vi "SubVI_ALD-Process_V16.vi"(0 "error in (no error)":errorcluster, 1 "Precursors List (Strings)":string[](array[string]), 2 "Digital Output Assignments":T7, 5 "output cluster":T3, 7 "output cluster 4":T2, 9 "Graph Ref Cluster":T4, 12 "Exec Array":dbl[][](array[numeric])) -> (4 "error out":errorcluster)   [LabVIEW 2026]
uses:
  <vilib>/Utility/miscctls.llb/LVRowAndColumnTypeDef.ctl
  <vilib>/Analysis/NI_AALBase.lvlib
  <vilib>/Analysis/baseanly.llb/Mean (DBL).vi
  CTRL_DO Boolean Array Cluster_V16.ctl
  CTRL_DO Arrays Precursor Process_V16.ctl
  CTRL_Digital-Out-Assignments_V16.ctl
panel:
  out "Total Steps":i32
  out "Summary File Refnum":refnum<file>
  in  "ProcessStep Input Cluster":T1
  out "DeltaM-i":dbl
  out "FinalMass-i":dbl
  out "InitialMass-i":dbl
  out "Dose File Refnum":refnum<file>
  out "Precursor-i name":string
  out "PrecursorValveArrays-i":T5
  out "ProcessType-i":i32
  out "PurgeTime-i":dbl
  out "DoseTime-i":dbl
  out "FillPressure-i":dbl
  out "Precursor-i":i32
  out "Delay Start Time (sec)":dbl
  out "ALD Running?":bool
  # "This VI receives the execution array and the reference cluster from the main VI to execute the ALD process. The VI first initilizes the valves to OFF, wait for the initial delay, then the VI processes the Execution Array line  by line and color each line as it is being processed. For each line of the Execution array, the VI calls the  ALDPulsePurge.vi if the Fill pressure is -1. Otherwise the ALD FHP.vi is called. There are 2 Pulse Purge processes. The Full Flow Pulse Purge process is used when the Pulse Purge Type control from the main VI is false, which indicates the Full Flow state. The Diversion Pulse Purge process is used when the Pulse Purge Type control is true. Finally, the VI returns the controls from the main VI to its original states."
  # "Module 7 Connections\nDigital Output (6V-30V)\n\n0:  Hold/Divert N2\n1:  Hold/Divert Manifold A\n2:  Hold/Divert Manifold B\n3:  Hold/Divert Manifold C\n4:  Hold/Divert Manifold D\n5:  Unused\n6:  Unused\n7:  Unused\n8:   V+ from 24V Power Supply\n9:   V- from 24V Power Supply"
  # "Module 8 Connections\nDigital Output (6V-30V)\n\n0:   Hold Chamber\n1:   Pulse A1\n2:   Pulse B1\n3:   Pulse C2\n4:   Pulse D2\n5:   Unused\n6:   Unused\n7:   Unused\n8:   V+ from 24V Power Supply\n9:   V- from 24V Power Supply"
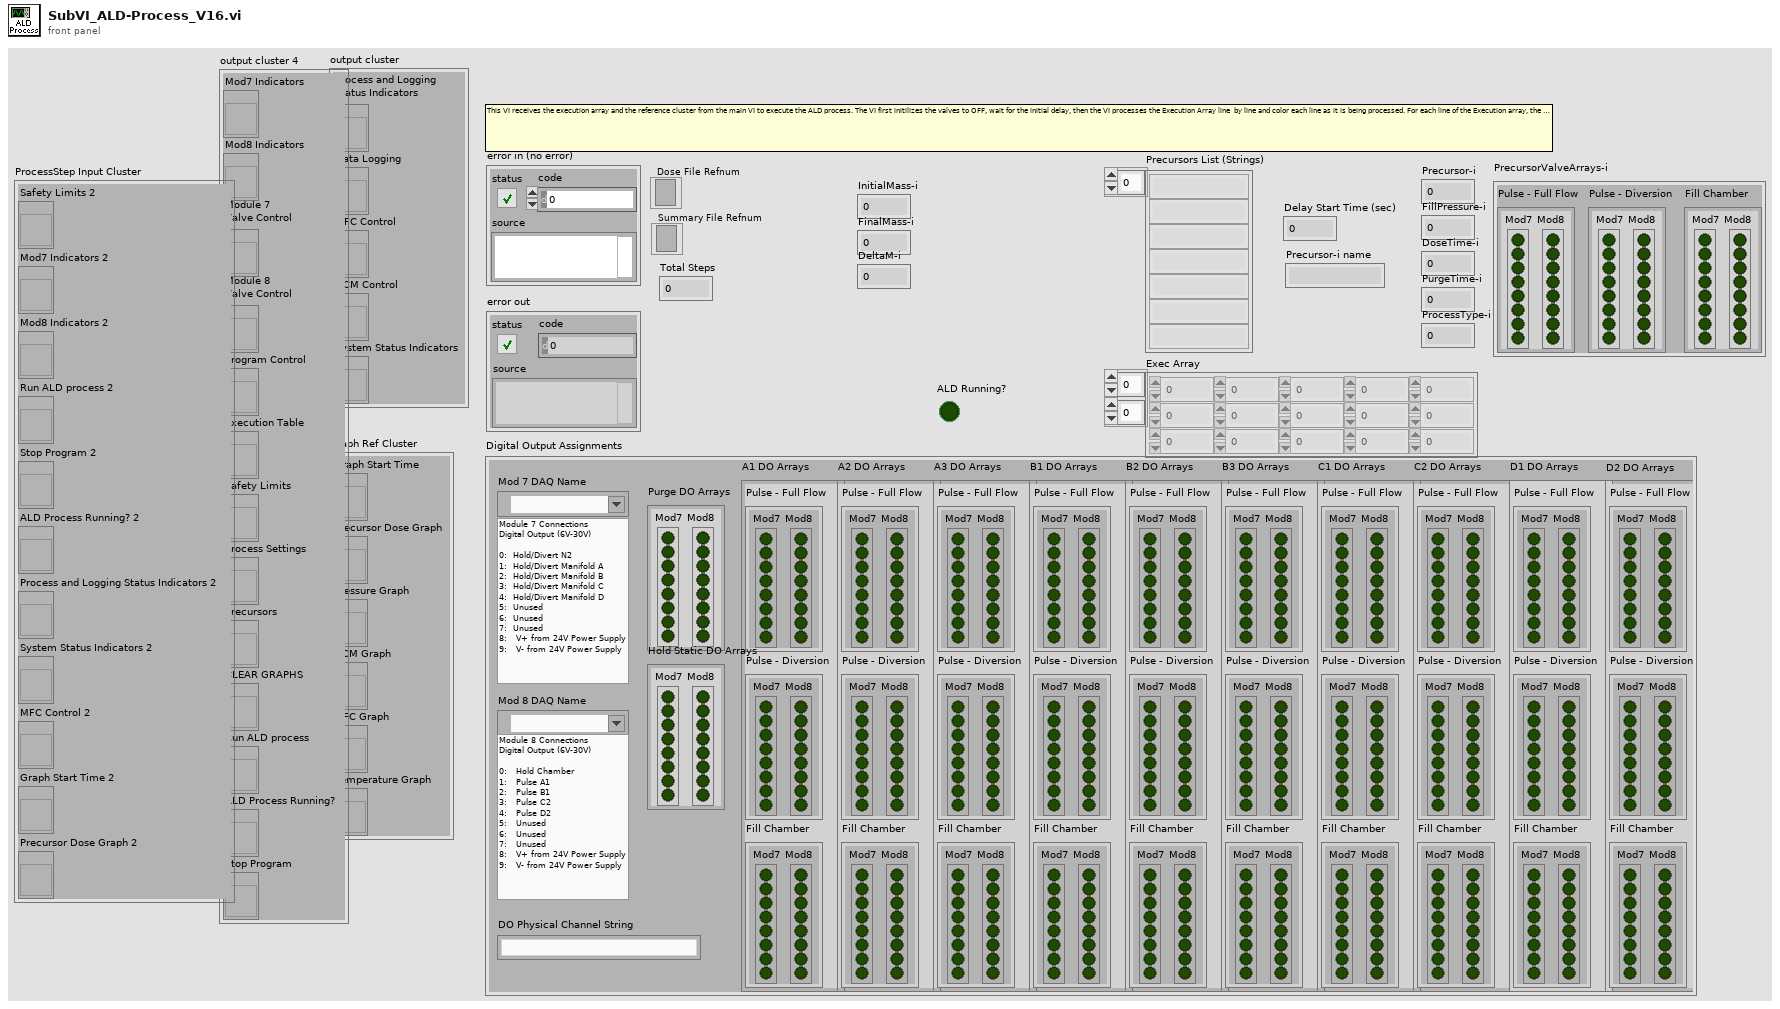
[diagram p1: front panel]
types:
  T1 = cluster{"Safety Limits 2":refnum<vi>, "Mod7 Indicators 2":refnum<vi>, "Mod8 Indicators 2":refnum<vi>, "Run ALD process 2":refnum<vi>, "Stop Program 2":refnum<vi>, "ALD Process Running? 2":refnum<vi>, "Process and Logging Status Indicators 2":refnum<vi>, "System Status Indicators 2":refnum<vi>, "MFC Control 2":refnum<vi>, "Graph Start Time 2":refnum<vi>, "Precursor Dose Graph 2":refnum<vi>}
  T2 = cluster{"Mod7 Indicators ":refnum<vi>, "Mod8 Indicators":refnum<vi>, "Module 7 \nValve Control":refnum<vi>, "Module 8 \nValve Control":refnum<vi>, "Program Control":refnum<vi>, "Execution Table":refnum<vi>, "Safety Limits":refnum<vi>, "Process Settings":refnum<vi>, "Precursors":refnum<vi>, "CLEAR GRAPHS":refnum<vi>, "Run ALD process":refnum<vi>, "ALD Process Running?":refnum<vi>, "Stop Program":refnum<vi>}
  T3 = cluster{"Process and Logging \nStatus Indicators":refnum<vi>, "Data Logging":refnum<vi>, "MFC Control":refnum<vi>, "QCM Control":refnum<vi>, "System Status Indicators":refnum<vi>}
  T4 = cluster{"Graph Start Time":refnum<vi>, "Precursor Dose Graph":refnum<vi>, "Pressure Graph":refnum<vi>, "QCM Graph":refnum<vi>, "MFC Graph":refnum<vi>, "Temperature Graph":refnum<vi>}
  T5 = typedef "CTRL_DO Arrays Precursor Process_V16.ctl" = cluster{"Pulse - Full Flow":T6, "Pulse - Diversion":T6, "Fill Chamber":T6}
  T6 = typedef "CTRL_DO Boolean Array Cluster_V16.ctl" = cluster{"Mod7":bool[], "Mod8":bool[]}
  T7 = typedef "CTRL_Digital-Out-Assignments_V16.ctl" = cluster{"Mod 7 DAQ Name":tag, "Mod 8 DAQ Name":tag, "DO Physical Channel String":string, "Purge DO Arrays":T6, "Hold Static DO Arrays":T6, "A1 DO Arrays":T5, "A2 DO Arrays":T5, "A3 DO Arrays":T5, "B1 DO Arrays":T5, "B2 DO Arrays":T5, "B3 DO Arrays":T5, "C1 DO Arrays":T5, "C2 DO Arrays":T5, "D1 DO Arrays":T5, "D2 DO Arrays":T5}
  T8 = typedef "LVRowAndColumnTypeDef.ctl" = cluster{"Row":i32, "Column":i32}
  T9 = enum16{"open", "replace", "create", "open or create", "replace or create", "replace or create with confirmation"}
  T10 = cluster{"Line 1":bool, "Line 2":bool, "Line 3":bool, "Line 4":bool, "Line 0":bool}
  T11 = cluster{"Data Log On?":bool, "User:":string, "Furnace Temp [ºC]":dbl, "Parent Directory:":path, "File Name Format:":string, "Notes:":string}
  T12 = typedef "System Status Indicators.ctl" = cluster{"System Status:":string, "Thermocouple 1":dbl, "Thermocouple 2":dbl, "Thermocouple 3":dbl, "Thermocouple 4":dbl, "Chamber Pressure (Torr)":dbl, "Pump Pressure (Torr)":dbl}
  T13 = cluster{"ALD Process Status:":string, "Logging Data to:":path, "Process Start Time:":string, "Process End Time:":string, "Steps Completed:":string}
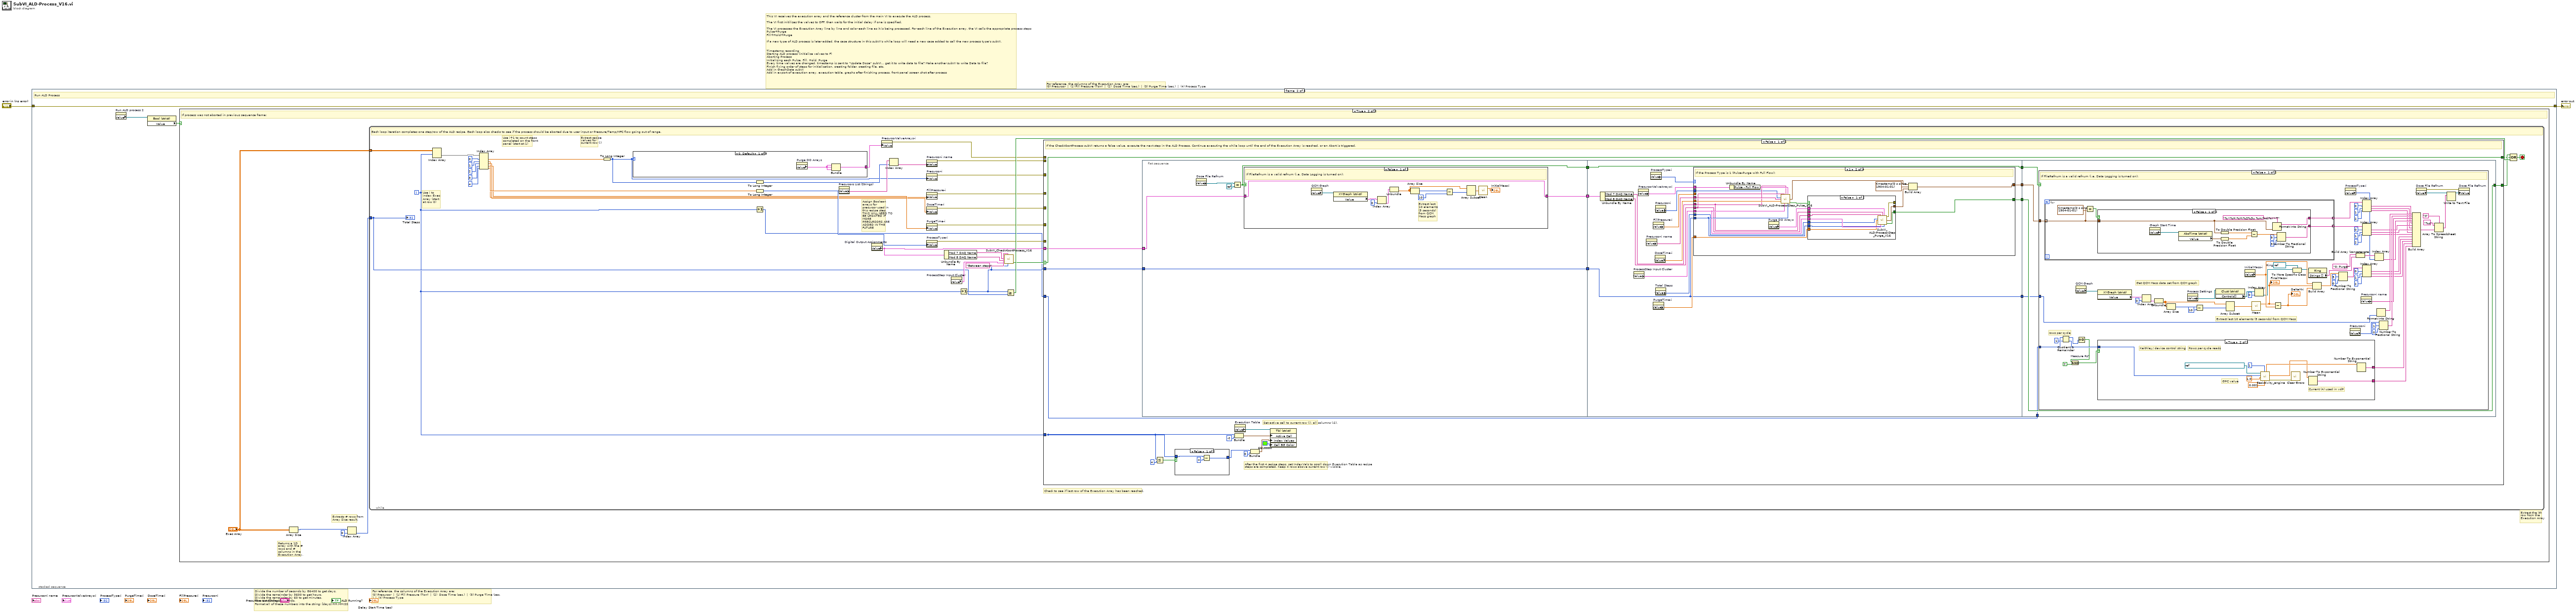
[diagram p0: block diagram]
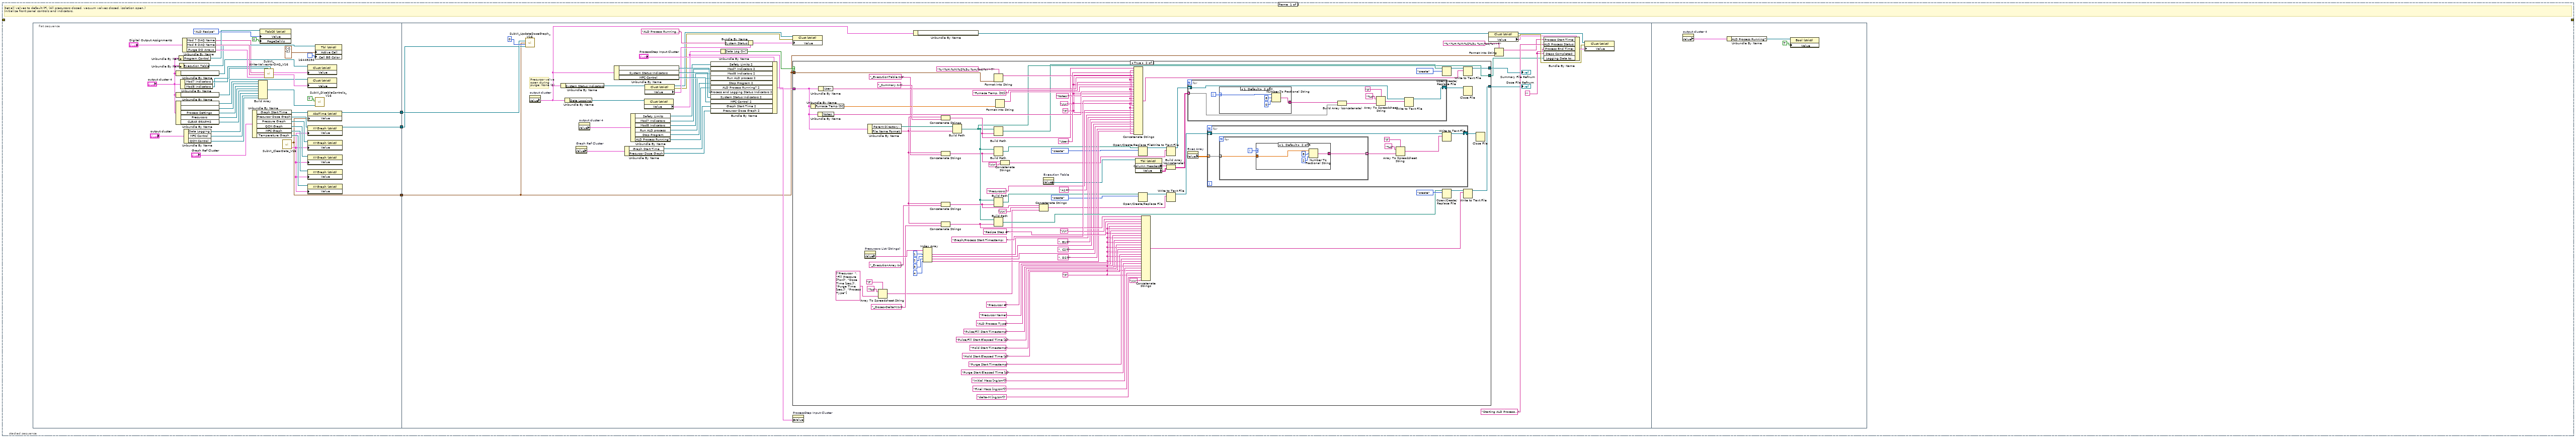
[diagram p2: hidden frame]
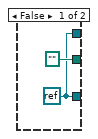
[diagram p3: hidden frame]
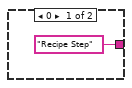
[diagram p4: hidden frame]
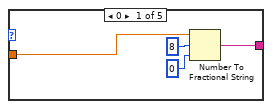
[diagram p5: hidden frame]
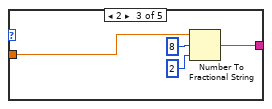
[diagram p6: hidden frame]
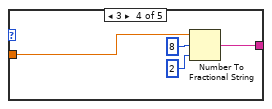
[diagram p7: hidden frame]
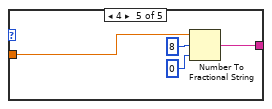
[diagram p8: hidden frame]
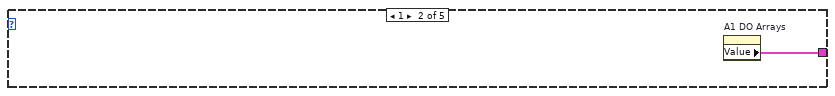
[diagram p10: hidden frame]
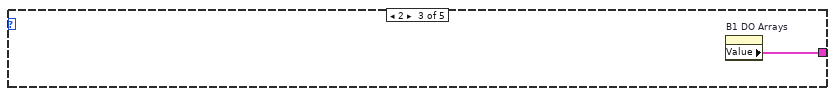
[diagram p11: hidden frame]
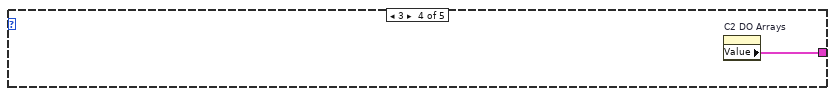
[diagram p12: hidden frame]
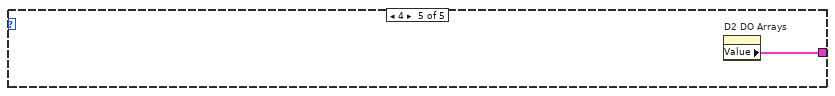
[diagram p13: hidden frame]
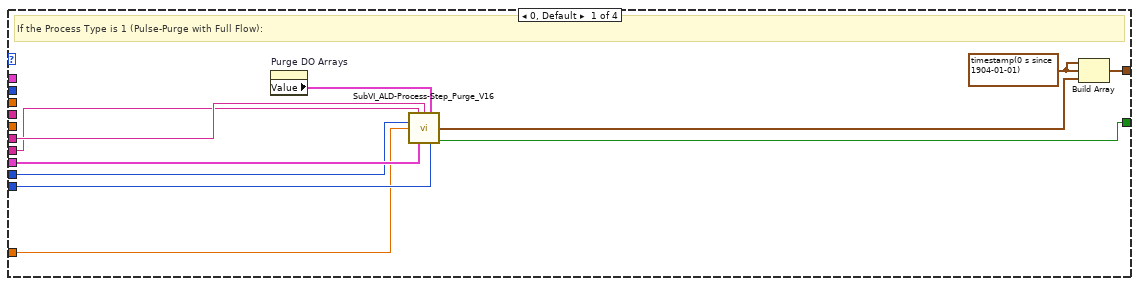
[diagram p15: hidden frame]
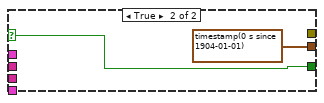
[diagram p16: hidden frame]
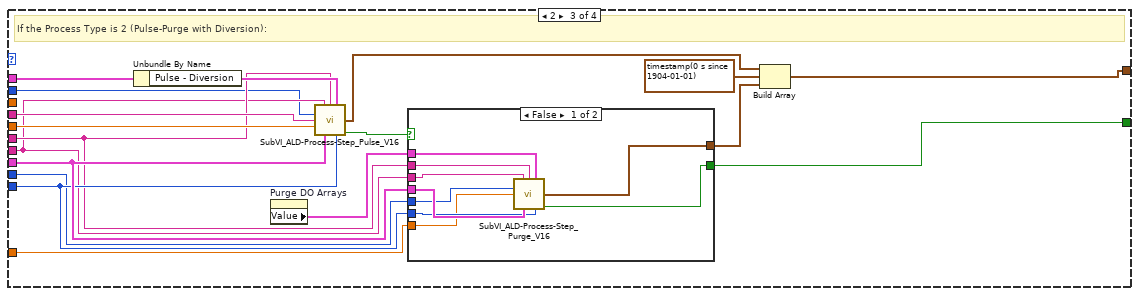
[diagram p17: hidden frame]
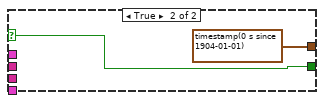
[diagram p18: hidden frame]
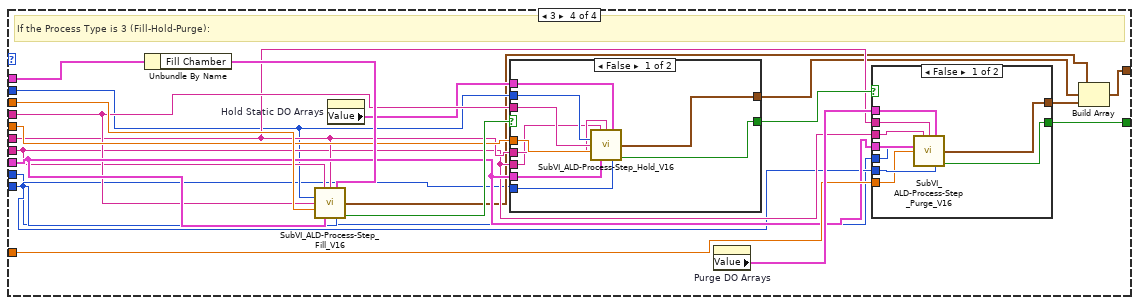
[diagram p19: hidden frame]
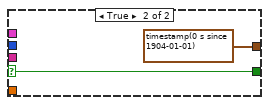
[diagram p20: hidden frame]
diagram:
  # "For reference, the columns of the Execution Array are:\n(0) Precursor  |  (1) Fill Pressure (Torr)  |  (2)  Dose Time (sec.)  |  (3) Purge Time (sec.)  |  (4) Process Type"
  # "For reference, the columns of the Execution Array are:\n(0) Precursor  |  (1) Fill Pressure (Torr)  |  (2)  Dose Time (sec.)  |  (3) Purge Time (sec.)  |  (4) Process Type"
  # "Divide the number of seconds by 86400 to get days.\nDivide the remainder by 3600 to get hours.\nDivide the remainder by 60 to get minutes.\nThe remainder is seconds.\nFormat all of these numbers into the string: [days] HH:MM:SS"
  # "This VI receives the execution array and the reference cluster from the main VI to execute the ALD process.\n\nThe VI first initilizes the valves to OFF, then waits for the initial delay if one is specified.\n\nThe VI processes the Execution Array line by line and color each line as it is being processed. For each line of the Execution array, the VI calls the appropriate process steps\nPulse+Purge\nFill+Hold+Purge\n\nIf a new type of ALD process is later added, the case structure in this subVI's while loop will need a new case added to call the new process type's subVI.\n\n\nTimestamp recording\nStarting ALD process (initialize valves to F)\nAborting Process\nInitializing each Pulse, Fill, Hold, Purge\nEvery time valves are changed, timestamp is sent to \"Update Dose\" subVI… get it to write data to file? Make another subVI to write Data to file?\nFinish fixing order of steps for initialization, creating folder, creating file, etc.\nAdd in GraphData subVI\nAdd in export of execution array, execution table, graphs after finishing process, front panel screen shot after process"
  n1 = stacked-sequence {
    tunnel: "error in (no error)" -> [_ w223 _]
    tunnel: [_ w223 _] -> w1
    frame #0 {
      # "Set all valves to default (F). (All precursors closed, vacuum valves closed, isolation open.)\nInitialize front panel controls and indicators."
      n2 = flat-sequence {
        tunnel: [w10] -> w5
        tunnel: [w9] -> w4
        tunnel: [w7] -> w3
        tunnel: w5 -> [w51]
        tunnel: w4 -> [w50]
        tunnel: w3 -> [w45]
        frame #0 {
          n3 = Unbundle By Name("output cluster 4") -> ("Module 7 \nValve Control"=w14:refnum<vi>)
          n4 = Unbundle By Name("output cluster 4") -> ("Module 8 \nValve Control"=w13:refnum<vi>)
          n5 = Unbundle By Name("output cluster 4") -> ("Module 7 \nValve Control"=w26:refnum<vi>, "Module 8 \nValve Control"=w25:refnum<vi>, "Process Settings"=w24:refnum<vi>, "Precursors"=w23:refnum<vi>, "CLEAR GRAPHS"=w22:refnum<vi>)
          n6 = Unbundle By Name("output cluster 4") -> ("Program Control"=w15:refnum<vi>)
          n7 = Unbundle By Name("output cluster 4") -> ("Execution Table"=w12:refnum<vi>)
          n8 = Unbundle By Name("output cluster 4") -> ("Mod7 Indicators"=w36:refnum<vi>, "Mod8 Indicators"=w35:refnum<vi>)
          n9 = Unbundle By Name("Digital Output Assignments") -> ("Mod 7 DAQ Name"=w6:tag, "Mod 8 DAQ Name"=w39:tag, "Purge DO Arrays"=w40:T6)
          n10 = Unbundle By Name("output cluster") -> ("Data Logging"=w21:refnum<vi>, "MFC Control"=w20:refnum<vi>, "QCM Control"=w19:refnum<vi>)
          n11 = Unbundle By Name("Graph Ref Cluster") -> ("Graph Start Time"=w34:refnum<vi>, "Precursor Dose Graph"=w33:refnum<vi>, "Pressure Graph"=w32:refnum<vi>, "QCM Graph"=w31:refnum<vi>, "MFC Graph"=w30:refnum<vi>, "Temperature Graph"=w29:refnum<vi>)
          n12 = Build Array(w26, w25, w24, w23, w22, w21, w20, w19) -> (w27:refnum<vi>[])
          n13 = property on="Property Node" class="TabCtl (strict)"(reference=w15, "Value"=enum32{"Initialization", "ALD Recipe"}."ALD Recipe", "PageSelVis"=TRUE ("Page Selector Visible")) -> ()  [unwired: 1 in, 2 out]
          n14 = call "SubVI_Write-Valves-to-DAQ_V16.vi"("Mod7 Indicators Ref"=w36, "Mod8 Indicators Ref"=w35, "DO Boolean Array Cluster"=w40, "Mod8 Port Name"=w39, "Mod7 Port Name"=w6) -> ("Mod8 Buttons"=w16:T10, "Mod7 Buttons"=w17:T10)  [unwired: 3 in, 2 out]
          n15 = call "SubVI_ClearData_V16.vi"() -> ("Time Stamp"=w7:timestamp, "Empty Graph Data"=w8:cluster{dbl[], dbl[]}[])  [unwired: 11 in, 3 out]
          n16 = property class="Clust (strict)"(reference=w14, "Value"=w17) -> ()  [unwired: 1 in, 2 out]
          n17 = property class="Clust (strict)"(reference=w13, "Value"=w16) -> ()  [unwired: 1 in, 2 out]
          n18 = property class="XYGraph (strict)"(reference=w33, "Value"=w8) -> (reference out=w9:refnum<vi>)  [unwired: 1 in, 1 out]
          n19 = property class="XYGraph (strict)"(reference=w32, "Value"=w8) -> ()  [unwired: 1 in, 2 out]
          n20 = property class="XYGraph (strict)"(reference=w31, "Value"=w8) -> ()  [unwired: 1 in, 2 out]
          n21 = property class="XYGraph (strict)"(reference=w30, "Value"=w8) -> ()  [unwired: 1 in, 2 out]
          n22 = property class="XYGraph (strict)"(reference=w29, "Value"=w8) -> ()  [unwired: 1 in, 2 out]
          n23 = property class="AbsTime (strict)"(reference=w34, "Value"=w7) -> (reference out=w10:refnum<vi>)  [unwired: 1 in, 1 out]
          n24 = property on="Property Node" class="Tbl (strict)"(reference=w12, "Active Cell"=T8 {"Row"=-2, "Column"=-2} ("Active Cell:Active Cell"), "Cell BG Color"=u32 16448250) -> ()  [unwired: 1 in, 2 out]
          n25 = call "SubVI_DisableControls_V16.vi"("appended array"=w27, "Disabled?"=TRUE) -> ()  [unwired: 9 in, 1 out]
        }
        frame #1 {
          w57 = ""
          # "Precursor valve open during purge: None (0)"
          n26 = call "SubVI_UpdateDoseGraph_V16.vi"("Graph Start Time"=w51, "New Timestamp"=w45, "Precursor Valve Open"=0 ("Precursor"), "Precursor Dose Graph"=w50) -> ()  [unwired: 11 in, 1 out]
          n27 = property on="output cluster" class="Clust (strict)"() -> ("Value"=w85:T3)  [unwired: 2 in, 2 out]
          n28 = Unbundle By Name(w85) -> ("System Status Indicators"=w55:refnum<vi>)
          n29 = Unbundle By Name(w85) -> ("Data Logging"=w68:refnum<vi>)
          n30 = property on="Graph Ref Cluster" class="Clust (strict)"() -> ("Value"=w76:T4)  [unwired: 2 in, 2 out]
          n31 = property on="output cluster 4" class="Clust (strict)"() -> ("Value"=w72:T2)  [unwired: 2 in, 2 out]
          n32 = Unbundle By Name(w85) -> ("Process and Logging \nStatus Indicators"=w80:refnum<vi>, "System Status Indicators"=w81:refnum<vi>, "MFC Control"=w82:refnum<vi>)
          n33 = Unbundle By Name(w76) -> ("Graph Start Time"=w83:refnum<vi>, "Precursor Dose Graph"=w84:refnum<vi>)
          n34 = Unbundle By Name(w72) -> ("Safety Limits"=w73:refnum<vi>, "Mod7 Indicators"=w74:refnum<vi>, "Mod8 Indicators"=w75:refnum<vi>, "Run ALD process"=w77:refnum<vi>, "Stop Program"=w78:refnum<vi>, "ALD Process Running?"=w79:refnum<vi>)
          n35 = property class="Clust (strict)"(reference=w68) -> ("Value"=w69:T11)  [unwired: 1 in, 2 out]
          n36 = property class="Clust (strict)"(reference=w55) -> (reference out=w65:refnum<vi>, error out=w64:errorcluster, "Value"=w67:T12)  [unwired: 1 in]
          n37 = Bundle By Name(cluster="ProcessStep Input Cluster", "Safety Limits 2"=w73, "Mod7 Indicators 2"=w74, "Mod8 Indicators 2"=w75, "Run ALD process 2"=w77, "Stop Program 2"=w78, "ALD Process Running? 2"=w79, "Process and Logging Status Indicators 2"=w80, "System Status Indicators 2"=w81, "MFC Control 2"=w82, "Graph Start Time 2"=w83, "Precursor Dose Graph 2"=w84) -> (w71:T1)
          n38 = Unbundle By Name(w69) -> ("Data Log On?"=w52:bool)
          n39 = Bundle By Name(cluster=w67, "System Status:"="ALD Process Running...") -> (w63:T12)
          n40 = property class="Clust (strict)"(reference=w65, error in=w64, "Value"=w63) -> ()  [unwired: 2 out]
          n41 = case shown="True" w52 {
            tunnel: [w86 w160] -> w53
            tunnel: w69 -> [_ w161]
            tunnel: w45 -> [_ w156]
            tunnel: [path "" w99] -> w48
            tunnel: [w86 w123] -> w49
            frame False {
              w86 = refnum<k0> refnum
            }
            frame True {
              w118 = "\t"
              w133 = "\t"
              w124 = "\r\n"
              n42 = Unbundle By Name(w161) -> ("Furnace Temp [ºC]"=w166:dbl)
              n43 = Unbundle By Name(w161) -> ("Notes:"=w165:string)
              n44 = Unbundle By Name(w161) -> ("User:"=w170:string)
              n45 = property on="Precursors List (Strings)" class="Arr (strict)"() -> ("Value"=w154:string[])  [unwired: 2 in, 2 out]
              n46 = Unbundle By Name(w161) -> ("Parent Directory:"=w155:path, "File Name Format:"=w98:string)
              n47 = Array To Spreadsheet String(delimiter (Tab)="\t", array=string[] ["Precursor  ", "Fill Pressure [Torr]", "Dose Time [sec.]", "Purge Time [sec.]", "Process Type"], 3:"%s" ("format string")) -> (spreadsheet string=w104:string)
              n48 = Index Array(array=w154, index #1=1 ("index"), index #2=2 ("index"), index #3=3 ("index"), index #4=4 ("index")) -> (element #1=w131:string, element #2=w129:string, element #3=w127:string, element #4=w126:string)
              n49 = Concatenate Strings(w98, "_Summary.txt" ("string")) -> (w119:string)
              n50 = Concatenate Strings(w98, "_ExecutionTable.txt" ("string")) -> (w90:string)
              n51 = Concatenate Strings(w98, "_ExecutionArray.txt" ("string")) -> (w109:string)
              n52 = Concatenate Strings(w98, "_Doses-DeltaM.txt" ("string")) -> (w136:string)
              n53 = Build Path(base path=w155, name or relative path=w98) -> (appended path=w99:path)
              n54 = Format Into String(format string="%<%H:%M:%S%3u %m/%d/%Y>T", w156) -> (resulting string=w163:string)  [unwired: 2 in, 1 out]
              n55 = Build Path(base path=w99, name or relative path=w119) -> (appended path=w139:path)
              n56 = Build Path(base path=w99, name or relative path=w90) -> (appended path=w100:path)
              n57 = Build Path(base path=w99, name or relative path=w109) -> (appended path=w115:path)
              n58 = Build Path(base path=w99, name or relative path=w136) -> (appended path=w162:path)
              n59 = Format Into String(w166) -> (resulting string=w168:string)  [unwired: 3 in, 1 out]
              n60 = Concatenate Strings(w90, "\r\n") -> (w88:string)
              n61 = Concatenate Strings(w109, "\r\n", w104) -> (w107:string)
              n62 = property on="Execution Table" class="LVObjRef (strict)"() -> ("Value"=w102:refnum<vi>)  [unwired: 2 in, 2 out]
              n63 = Concatenate Strings(w119, w124, "User:", w133, w170, w124, "Furnace Temp. [ºC]:", w133, w168, w124, "Notes:", w133, w165, w124, "Graph/Process Start Timestamp:   ", w133, w163, w124, "Precursors:", w133, "A1=", w131, ", B1=", w129, ", C2=", w127, ", D2=", w126, w124) -> (w121:string)
              n64 = property class="Tbl (strict)"(reference=w102) -> ("Column Headers[]"=w93:string[], "Value"=w92:string[][])  [unwired: 1 in, 2 out]
              n65 = Open/Create/Replace File(file path (use dialog)=w100, operation (0:open)=T9."create") -> (refnum out=w101:refnum<file>)  [unwired: 4 in, 2 out]
              n66 = Open/Create/Replace File(file path (use dialog)=w115, operation (0:open)=T9."create") -> (refnum out=w111:refnum<file>)  [unwired: 4 in, 2 out]
              n67 = Concatenate Strings(w136, "\r\n", "Recipe Step #", w118, "Precursor #", w118, "Precursor Name", w118, "ALD Process Type", w118, "Pulse/Fill Start Timestamp", w118, "Pulse/Fill Start Elapsed Time [s]", w118, "Hold Start Timestamp", w118, "Hold Start Elapsed Time [s]", w118, "Purge Start Timestamp", w118, "Purge Start Elapsed Time [s]", w118, "Initial Mass [ng/cm²]", w118, "Final Mass [ng/cm²]", w118, "delta-M [ng/cm²]", "\r\n") -> (w135:string)
              n68 = Write to Text File(file (use dialog)=w101, text=w88) -> (refnum out=w95:refnum<file>)  [unwired: 2 in, 2 out]
              n69 = Build Array (concatenate)(w93, w92) -> (w91:string[][])
              n70 = Write to Text File(file (use dialog)=w111, text=w107) -> (refnum out=w110:refnum<file>)  [unwired: 2 in, 2 out]
              n71 = for {
                shift-right: [w179] -> w94
                shift-left: w95 -> [w180]
                tunnel: w91 -> [w178] mode=indexing
                i -> [w177]
                n72 = case shown="1, Default" w177 {
                  selector: w177 -> [_ w189]
                  tunnel: ["Recipe Step" ("format string") w186] -> w184
                  frame 0 {
                  }
                  frame 1, Default {
                    n73 = Number To Fractional String(number=w189, width (-)=i16 8, precision (6)=i16 0) -> (F-format string=w186:string)  [unwired: 1 in]
                  }
                }
                n74 = Build Array (concatenate)(w184, w178) -> (w176:string[])
                n75 = Array To Spreadsheet String(delimiter (Tab)="\t", array=w176, 3:"%s" ("format string")) -> (spreadsheet string=w183:string)
                n76 = Write to Text File(file (use dialog)=w180, text=w183) -> (refnum out=w179:refnum<file>)  [unwired: 2 in, 2 out]
              }
              n77 = property on="Exec Array" class="Arr (strict)"() -> ("Value"=w113:dbl[][])  [unwired: 2 in, 2 out]
              n78 = for {
                tunnel: w113 -> [w190] mode=indexing
                shift-right: [w191] -> w112
                shift-left: w110 -> [w194]
                n79 = for {
                  tunnel: [w198] -> w196 mode=indexing
                  tunnel: w190 -> [w197] mode=indexing
                  i -> [w199]
                  n80 = case shown="1, Default" w199 {
                    tunnel: w197 -> [w203 w207 w211 w215 w219]
                    tunnel: [w200 w204 w208 w212 w216] -> w198
                    frame 0 {
                      n81 = Number To Fractional String(number=w203, width (-)=i16 8, precision (6)=i16 0) -> (F-format string=w200:string)  [unwired: 1 in]
                    }
                    frame 1, Default {
                      n82 = Number To Fractional String(number=w207, width (-)=i16 8, precision (6)=i16 2) -> (F-format string=w204:string)  [unwired: 1 in]
                    }
                    frame 2 {
                      n83 = Number To Fractional String(number=w211, width (-)=i16 8, precision (6)=i16 2) -> (F-format string=w208:string)  [unwired: 1 in]
                    }
                    frame 3 {
                      n84 = Number To Fractional String(number=w215, width (-)=i16 8, precision (6)=i16 2) -> (F-format string=w212:string)  [unwired: 1 in]
                    }
                    frame 4 {
                      n85 = Number To Fractional String(number=w219, width (-)=i16 8, precision (6)=i16 0) -> (F-format string=w216:string)  [unwired: 1 in]
                    }
                  }
                }
                n86 = Array To Spreadsheet String(delimiter (Tab)="\t", array=w196, 3:"%s" ("format string")) -> (spreadsheet string=w192:string)
                n87 = Write to Text File(file (use dialog)=w194, text=w192) -> (refnum out=w191:refnum<file>)  [unwired: 2 in, 2 out]
              }
              n88 = Open/Create/Replace File(file path (use dialog)=w139, operation (0:open)=T9."create") -> (refnum out=w122:refnum<file>)  [unwired: 4 in, 2 out]
              n89 = Open/Create/Replace File(file path (use dialog)=w162, operation (0:open)=T9."create") -> (refnum out=w173:refnum<file>)  [unwired: 4 in, 2 out]
              n90 = Write to Text File(file (use dialog)=w122, text=w121) -> (refnum out=w123:refnum<file>)  [unwired: 2 in, 2 out]
              n91 = Close File(refnum=w94) -> ()  [unwired: 1 in, 2 out]
              n92 = Write to Text File(file (use dialog)=w173, text=w135) -> (refnum out=w160:refnum<file>)  [unwired: 2 in, 2 out]
              n93 = Close File(refnum=w112) -> ()  [unwired: 1 in, 2 out]
            }
          }
          "Dose File Refnum" <- w53
          "Summary File Refnum" <- w49
          n94 = property on="ProcessStep Input Cluster" class="Clust (strict)"("Value"=w71) -> ()  [unwired: 2 in, 2 out]
          n95 = Unbundle By Name(w85) -> ("Process and Logging \nStatus Indicators"=w54:refnum<vi>)
          n96 = property class="Clust (strict)"(reference=w54) -> (reference out=w60:refnum<vi>, error out=w61:errorcluster, "Value"=w59:T13)  [unwired: 1 in]
          n97 = Format Into String(format string="%<%H:%M:%S%3u %m/%d/%Y>T", w45) -> (resulting string=w46:string)  [unwired: 2 in, 1 out]
          n98 = Bundle By Name(cluster=w59, "Process Start Time:"=w46, "ALD Process Status:"="Starting ALD Process...", "Process End Time:"=w57, "Steps Completed:"=w57, "Logging Data to:"=w48) -> (w62:T13)
          n99 = property class="Clust (strict)"(reference=w60, error in=w61, "Value"=w62) -> ()  [unwired: 2 out]
        }
        frame #2 {
          n100 = property on="output cluster 4" class="Clust (strict)"() -> ("Value"=w220:T2)  [unwired: 2 in, 2 out]
          n101 = Unbundle By Name(w220) -> ("ALD Process Running?"=w222:refnum<vi>)
          n102 = property class="Bool (strict)"(reference=w222, "Value"=TRUE) -> ()  [unwired: 1 in, 2 out]
        }
      }
    }
    frame #1 {
      # "Run ALD Process"
      n103 = property on="Run ALD process 2" class="LVObjRef (strict)"() -> ("Value"=w225:refnum<vi>)  [unwired: 2 in, 2 out]
      n104 = property class="Bool (strict)"(reference=w225) -> ("Value"=w224:bool)  [unwired: 1 in, 2 out]
      n105 = case shown="True" w224 {
        frame False {
        }
        frame True {
          # "Extract the ith row from the Execution Array"
          # "Extracts # rows from Array Size result."
          # "Returns a 1D array with the # rows and # columns in the Execution Array."
          # "If process was not aborted in previous sequence frame:"
          n106 = Array Size(array="Exec Array") -> (size(s)=w227:i32[])
          n107 = Index Array(array=w227, index=0) -> (element=w226:i32)
          n108 = while {
            tunnel: "Exec Array" -> [w262]
            tunnel: w226 -> [w232]
            i -> [w231]
            stop <- w265 stop-if-true
            # "Use i+1 to count steps completed on the front panel (start at 1)"
            # "Use i to index Exec Array (start at row 0)"
            # "Assign Boolean arrays for precursor used in this recipe step.\nTHIS WILL NEED TO BE UPDATED IF MORE PRECURSORS ARE ADDED IN THE FUTURE"
            # "Extract recipe values for current row (i)"
            # "Check to see if last row of the Execution Array has been reached."
            # "Each loop iteration completes one step/row of the ALD recipe. Each loop also checks to see if the process should be aborted due to user input or Pressure/Temp/MFC flow going out of range."
            n109 = Index Array(array=w262, index (row)=w231) -> (element=w248:dbl[])  [unwired: 1 in]
            n110 = Index Array(array=w248, index #1=0 ("index"), index #2=1 ("index"), index #3=2 ("index"), index #4=3 ("index"), index #5=4 ("index")) -> (element #1=w258:dbl, element #2=w254:dbl, element #3=w255:dbl, element #4=w256:dbl, element #5=w257:dbl)
            n111 = To Long Integer(number=w258) -> (32bit integer=w247:i32)
            n112 = case shown="0, Default" w247 {
              tunnel: [w269 w271 w272 w273 w274] -> w246
              frame 0, Default {
                n113 = property on="Purge DO Arrays" class="Clust (strict)"() -> ("Value"=w270:T6)  [unwired: 2 in, 2 out]
                n114 = Bundle("Value"=w270, "Value"=w270, "Value"=w270) -> (w269:cluster{"Value":T6, "Value":T6, "Value":T6})  [unwired: 1 in]
              }
              frame 1 {
                n115 = property on="A1 DO Arrays" class="Clust (strict)"() -> ("Value"=w271:T5)  [unwired: 2 in, 2 out]
              }
              frame 2 {
                n116 = property on="B1 DO Arrays" class="Clust (strict)"() -> ("Value"=w272:T5)  [unwired: 2 in, 2 out]
              }
              frame 3 {
                n117 = property on="C2 DO Arrays" class="Clust (strict)"() -> ("Value"=w273:T5)  [unwired: 2 in, 2 out]
              }
              frame 4 {
                n118 = property on="D2 DO Arrays" class="Clust (strict)"() -> ("Value"=w274:T5)  [unwired: 2 in, 2 out]
              }
            }
            n119 = To Long Integer(number=w247) -> (32bit integer=w259:i32)
            n120 = To Long Integer(number=w257) -> (32bit integer=w261:i32)
            n121 = Increment(x=w231) -> (x+1=w230:i32)
            n122 = property on="Precursors List (Strings)" class="Arr (strict)"() -> ("Value"=w260:string[])  [unwired: 2 in, 2 out]
            n123 = property on="Digital Output Assignments" class="Clust (strict)"() -> ("Value"=w234:T7)  [unwired: 2 in, 2 out]
            n124 = property on="PrecursorValveArrays-i" class="Clust (strict)"("Value"=w246) -> (error out=w243:errorcluster)  [unwired: 2 in, 1 out]
            n125 = Index Array(array=w260, index=w259) -> (element=w245:string)
            n126 = property on="Precursor-i name" class="Str"("Value"=w245) -> (error out=w244:errorcluster)  [unwired: 2 in, 1 out]
            n127 = property on="Precursor-i" class="DigNum (strict)"("Value"=w247) -> (error out=w242:errorcluster)  [unwired: 2 in, 1 out]
            n128 = property on="FillPressure-i" class="DigNum (strict)"("Value"=w254) -> (error out=w241:errorcluster)  [unwired: 2 in, 1 out]
            n129 = property on="DoseTime-i" class="DigNum (strict)"("Value"=w255) -> (error out=w240:errorcluster)  [unwired: 2 in, 1 out]
            n130 = property on="PurgeTime-i" class="DigNum (strict)"("Value"=w256) -> (error out=w239:errorcluster)  [unwired: 2 in, 1 out]
            n131 = property on="ProcessType-i" class="DigNum (strict)"("Value"=w261) -> (error out=w238:errorcluster)  [unwired: 2 in, 1 out]
            n132 = Unbundle By Name(w234) -> ("Mod 7 DAQ Name"=w235:tag, "Mod 8 DAQ Name"=w236:tag)
            n133 = property on="ProcessStep Input Cluster" class="Clust (strict)"() -> ("Value"=w237:T1)  [unwired: 2 in, 2 out]
            n134 = Increment(x=w231) -> (x+1=w233:i32)
            n135 = call "SubVI_CheckAbortProcess_V16.vi"("Process Step"=w233, "Step Description"="Between steps", "ProcessStep Input Cluster"=w237, "Mod8 DAQ Name"=w236, "Mod7 DAQ Name"=w235) -> ("Abort Process Execution"=w264:bool)  [unwired: 5 in, 1 out]
            n136 = Greater Or Equal?(x=w233, y=w232) -> (x >= y?=w268:bool)
            n137 = case shown="False" w264 {
              selector: w264 -> [w296 w553]
              tunnel: w231 -> [w287 _]
              tunnel: [w286 w553] -> w267
              tunnel: [w296 w553] -> w266
              tunnel: w244 -> [_ _]
              tunnel: w243 -> [_ _]
              tunnel: w242 -> [_ _]
              tunnel: w241 -> [_ _]
              tunnel: w240 -> [_ _]
              tunnel: w239 -> [_ _]
              tunnel: w238 -> [_ _]
              tunnel: w234 -> [w284 _]
              tunnel: w233 -> [w276 _]
              tunnel: w230 -> [w275 _]
              frame False {
                # "Set active cell to current row (i), all columns (-2)."
                # "After the first 4 recipe steps, set IndexVals to scroll down Execution Table as recipe steps are completed. Keep 4 rows above current row (i) visible."
                # "If the CheckAbortProcess subVI returns a false value, execute the next step in the ALD Process. Continue executing the while loop until the end of the Execution Array is reached, or an Abort is triggered."
                n138 = flat-sequence {
                  tunnel: w284 -> [w299]
                  tunnel: w276 -> [w302]
                  tunnel: [w302] -> w283
                  tunnel: [w298] -> w282
                  tunnel: [w297] -> w279
                  tunnel: w283 -> [w316]
                  tunnel: w282 -> [w321]
                  tunnel: [w326] -> w281
                  tunnel: [w318] -> w280
                  tunnel: w279 -> [w318]
                  tunnel: [w317] -> w278
                  tunnel: [w316] -> w277
                  tunnel: [w449] -> w286
                  tunnel: w281 -> [w449]
                  tunnel: w280 -> [w448]
                  tunnel: w278 -> [w447]
                  tunnel: w277 -> [w446]
                  tunnel: w275 -> [w445]
                  frame #0 {
                    n139 = property on="Dose File Refnum" class="Ref (strict)"() -> ("Value"=w301:refnum<file>)  [unwired: 2 in, 2 out]
                    n140 = Equal?(x=w301, y=refnum<k0> refnum) -> (x = y?=w297:bool)
                    n141 = case shown="False" w297 {
                      tunnel: w299 -> [w313 w314]
                      tunnel: [w313 w314] -> w298
                      frame False {
                        # "Extract last 10 elements (5 seconds) from QCM Mass graph"
                        # "If FileRefnum is a valid refnum (i.e. Data Logging is turned on):"
                        n142 = property on="QCM Graph" class="LVObjRef (strict)"() -> ("Value"=w312:refnum<vi>)  [unwired: 2 in, 2 out]
                        n143 = property class="XYGraph (strict)"(reference=w312) -> ("Value"=w311:cluster{dbl[], dbl[]}[])  [unwired: 1 in, 2 out]
                        n144 = Index Array(array=w311, index=0) -> (element=w309:cluster{dbl[], dbl[]})
                        n145 = Unbundle(w309) -> (w307:dbl[])  [unwired: 1 out]
                        n146 = Array Size(array=w307) -> (size(s)=w308:i32)
                        n147 = Subtract(x=w308, y=10) -> (x-y=w305:i32)
                        n148 = Array Subset(array=w307, index=w305) -> (w304:dbl[])  [unwired: 1 in]
                        n149 = call-poly <vilib>:"Mean.vi"("X"=w304) -> ("mean"=→"InitialMass-i":dbl)  [unwired: 1 out]
                      }
                      frame True {
                        # "If FileRefnum is not a refnum (i.e. Data Logging is off) do nothing"
                      }
                    }
                  }
                  frame #1 {
                    n150 = Unbundle By Name(w321) -> ("Mod 7 DAQ Name"=w320:tag, "Mod 8 DAQ Name"=w319:tag)
                    n151 = property on="ProcessStep Input Cluster" class="Clust (strict)"() -> ("Value"=w322:T1)  [unwired: 2 in, 2 out]
                    n152 = property on="PrecursorValveArrays-i" class="Clust (strict)"() -> ("Value"=w327:T5)  [unwired: 2 in, 2 out]
                    n153 = property on="Precursor-i name" class="Str"() -> ("Value"=w329:string)  [unwired: 2 in, 2 out]
                    n154 = property on="ProcessType-i" class="DigNum (strict)"() -> ("Value"=w330:i32)  [unwired: 2 in, 2 out]
                    n155 = property on="FillPressure-i" class="DigNum (strict)"() -> ("Value"=w324:dbl)  [unwired: 2 in, 2 out]
                    n156 = property on="PurgeTime-i" class="DigNum (strict)"() -> ("Value"=w325:dbl)  [unwired: 2 in, 2 out]
                    n157 = property on="DoseTime-i" class="DigNum (strict)"() -> ("Value"=w328:dbl)  [unwired: 2 in, 2 out]
                    n158 = property on="Precursor-i" class="DigNum (strict)"() -> ("Value"=w323:i32)  [unwired: 2 in, 2 out]
                    n159 = property on="Total Steps" class="DigNum (strict)"() -> ("Value"=w315:i32)  [unwired: 2 in, 2 out]
                    n160 = case shown="1" w330 {
                      tunnel: w322 -> [w340 w354 w384 w413]
                      tunnel: w329 -> [_ w358 w388 w411]
                      tunnel: w328 -> [_ w357 w387 w412]
                      tunnel: w316 -> [w339 w353 w383 w402]
                      tunnel: w327 -> [_ w356 w386 w420]
                      tunnel: [w338 w351 w381 w418] -> w326
                      tunnel: w325 -> [w337 w350 w380 w417]
                      tunnel: w324 -> [_ _ _ w415]
                      tunnel: w323 -> [_ w347 w377 w407]
                      tunnel: w320 -> [w336 w349 w379 w409]
                      tunnel: w319 -> [w335 w348 w378 w408]
                      tunnel: [w334 w344 w373 w406] -> w317
                      tunnel: w315 -> [w332 w342 w372 w401]
                      frame 0, Default {
                        w331 = timestamp(0 s since 1904-01-01)
                        # "If the Process Type is 1 (Pulse-Purge with Full Flow):"
                        n161 = property on="Purge DO Arrays" class="Clust (strict)"() -> ("Value"=w341:T6)  [unwired: 2 in, 2 out]
                        n162 = call "SubVI_ALD-Process-Step_Purge_V16.vi"("Mod8 DAQ Name"=w335, "Mod7 DAQ Name"=w336, "Purge Array"=w341, "Total # Steps"=w332, "Purge Time (sec)"=w337, "ProcessStep Input Cluster"=w340, "Recipe Step \nNumber"=w339) -> ("Purge Start Timestamp"=w333:timestamp, "Execution Aborted \nDuring This Recipe Step?"=w338:bool)  [unwired: 6 in, 1 out]
                        n163 = Build Array(w331, w331, w333) -> (w334:timestamp[])
                      }
                      frame 1 {
                        # "If the Process Type is 1 (Pulse-Purge with Full Flow):"
                        n164 = Unbundle By Name(w356) -> ("Pulse - Full Flow"=w359:T6)
                        n165 = property on="Purge DO Arrays" class="Clust (strict)"() -> ("Value"=w355:T6)  [unwired: 2 in, 2 out]
                        n166 = call "SubVI_ALD-Process-Step_Pulse_V16.vi"("Mod8 DAQ Name"=w348, "Mod7 DAQ Name"=w349, "Precursor Dose Array"=w359, "Precursor-i"=w347, "Precursor-i name"=w358, "Dose Time (sec)"=w357, "ProcessStep Input Cluster"=w354, "Recipe Step \nNumber"=w353) -> ("Dose Start Timestamp"=w346:timestamp, "Execution Aborted \nDuring This Recipe Step?"=w352:bool)  [unwired: 5 in, 1 out]
                        n167 = case shown="False" w352 {
                          selector: w352 -> [_ w371]
                          tunnel: w355 -> [w369 _]
                          tunnel: w354 -> [w368 _]
                          tunnel: w353 -> [w367 _]
                          tunnel: [w366 w371] -> w351
                          tunnel: w350 -> [w365 _]
                          tunnel: w349 -> [w364 _]
                          tunnel: w348 -> [w363 _]
                          tunnel: [w362 timestamp(0 s since 1904-01-01)] -> w343
                          tunnel: w342 -> [w361 _]
                          tunnel: [w360 _] -> _
                          frame False {
                            n168 = call "SubVI_ALD-Process-Step_Purge_V16.vi"("Mod8 DAQ Name"=w363, "Mod7 DAQ Name"=w364, "Purge Array"=w369, "Total # Steps"=w361, "Purge Time (sec)"=w365, "ProcessStep Input Cluster"=w368, "Recipe Step \nNumber"=w367) -> ("error out"=w360:errorcluster, "Purge Start Timestamp"=w362:timestamp, "Execution Aborted \nDuring This Recipe Step?"=w366:bool)  [unwired: 6 in]
                          }
                          frame True {
                          }
                        }
                        n169 = Build Array(w346, timestamp(0 s since 1904-01-01), w343) -> (w344:timestamp[])
                      }
                      frame 2 {
                        # "If the Process Type is 2 (Pulse-Purge with Diversion):"
                        n170 = Unbundle By Name(w386) -> ("Pulse - Diversion"=w389:T6)
                        n171 = property on="Purge DO Arrays" class="Clust (strict)"() -> ("Value"=w385:T6)  [unwired: 2 in, 2 out]
                        n172 = call "SubVI_ALD-Process-Step_Pulse_V16.vi"("Mod8 DAQ Name"=w378, "Mod7 DAQ Name"=w379, "Precursor Dose Array"=w389, "Precursor-i"=w377, "Precursor-i name"=w388, "Dose Time (sec)"=w387, "ProcessStep Input Cluster"=w384, "Recipe Step \nNumber"=w383) -> ("Dose Start Timestamp"=w376:timestamp, "Execution Aborted \nDuring This Recipe Step?"=w382:bool)  [unwired: 5 in, 1 out]
                        n173 = case shown="False" w382 {
                          selector: w382 -> [_ w400]
                          tunnel: w385 -> [w398 _]
                          tunnel: w384 -> [w397 _]
                          tunnel: w383 -> [w396 _]
                          tunnel: [w395 w400] -> w381
                          tunnel: w380 -> [w394 _]
                          tunnel: w379 -> [w393 _]
                          tunnel: w378 -> [w392 _]
                          tunnel: [w391 timestamp(0 s since 1904-01-01)] -> w375
                          tunnel: w372 -> [w390 _]
                          frame False {
                            n174 = call "SubVI_ALD-Process-Step_Purge_V16.vi"("Mod8 DAQ Name"=w392, "Mod7 DAQ Name"=w393, "Purge Array"=w398, "Total # Steps"=w390, "Purge Time (sec)"=w394, "ProcessStep Input Cluster"=w397, "Recipe Step \nNumber"=w396) -> ("Purge Start Timestamp"=w391:timestamp, "Execution Aborted \nDuring This Recipe Step?"=w395:bool)  [unwired: 6 in, 1 out]
                          }
                          frame True {
                          }
                        }
                        n175 = Build Array(w376, timestamp(0 s since 1904-01-01), w375) -> (w373:timestamp[])
                      }
                      frame 3 {
                        # "If the Process Type is 3 (Fill-Hold-Purge):"
                        n176 = Unbundle By Name(w420) -> ("Fill Chamber"=w421:T6)
                        n177 = call "SubVI_ALD-Process-Step_Fill_V16.vi"("Mod8 DAQ Name"=w408, "Mod7 DAQ Name"=w409, "Precursor Fill Array"=w421, "Precursor-i"=w407, "Precursor-i name"=w411, "Fill Pressure (Torr)"=w415, "ProcessStep Input Cluster"=w413, "Recipe Step \nNumber"=w402) -> ("Fill Start Timestamp"=w405:timestamp, "Execution Aborted \nDuring This Recipe Step?"=w414:bool)  [unwired: 5 in, 1 out]
                        n178 = property on="Hold Static DO Arrays" class="Clust (strict)"() -> ("Value"=w410:T6)  [unwired: 2 in, 2 out]
                        n179 = case shown="False" w414 {
                          selector: w414 -> [_ w433]
                          tunnel: w410 -> [w431 _]
                          tunnel: w413 -> [w430 _]
                          tunnel: w402 -> [w429 _]
                          tunnel: [w428 w433] -> w416
                          tunnel: w412 -> [w427 _]
                          tunnel: w407 -> [w426 _]
                          tunnel: w411 -> [w425 _]
                          tunnel: w409 -> [w424 _]
                          tunnel: w408 -> [w423 _]
                          tunnel: [w422 timestamp(0 s since 1904-01-01)] -> w404
                          frame False {
                            n180 = call "SubVI_ALD-Process-Step_Hold_V16.vi"("Mod8 DAQ Name"=w423, "Mod7 DAQ Name"=w424, "Hold Array"=w431, "Precursor-i"=w426, "Precursor-i name"=w425, "Hold Time (sec)"=w427, "ProcessStep Input Cluster"=w430, "Recipe Step \nNumber"=w429) -> ("Hold Start Timestamp"=w422:timestamp, "Execution Aborted \nDuring This Recipe Step?"=w428:bool)  [unwired: 5 in, 1 out]
                          }
                          frame True {
                          }
                        }
                        n181 = property on="Purge DO Arrays" class="Clust (strict)"() -> ("Value"=w419:T6)  [unwired: 2 in, 2 out]
                        n182 = case shown="False" w416 {
                          selector: w416 -> [_ w444]
                          tunnel: w419 -> [w442 _]
                          tunnel: w413 -> [w441 _]
                          tunnel: w402 -> [w440 _]
                          tunnel: [w439 w444] -> w418
                          tunnel: w417 -> [w438 _]
                          tunnel: w409 -> [w437 _]
                          tunnel: w408 -> [w436 _]
                          tunnel: [w435 timestamp(0 s since 1904-01-01)] -> w403
                          tunnel: w401 -> [w434 _]
                          frame False {
                            n183 = call "SubVI_ALD-Process-Step_Purge_V16.vi"("Mod8 DAQ Name"=w436, "Mod7 DAQ Name"=w437, "Purge Array"=w442, "Total # Steps"=w434, "Purge Time (sec)"=w438, "ProcessStep Input Cluster"=w441, "Recipe Step \nNumber"=w440) -> ("Purge Start Timestamp"=w435:timestamp, "Execution Aborted \nDuring This Recipe Step?"=w439:bool)  [unwired: 6 in, 1 out]
                          }
                          frame True {
                          }
                        }
                        n184 = Build Array(w405, w404, w403) -> (w406:timestamp[])
                      }
                    }
                  }
                  frame #2 {
                    n185 = case shown="False" w448 {
                      tunnel: w446 -> [w511 _]
                      tunnel: w447 -> [w510 _]
                      tunnel: w445 -> [w456 _]
                      frame False {
                        w478 = refnum<vi> refnum  # Ring
                        # "rows per cycle"
                        # "Get QCM Mass data set from QCM graph"
                        # "Extract last 10 elements (5 seconds) from QCM Mass"
                        # "If FileRefnum is a valid refnum (i.e. Data Logging is turned on):"
                        n186 = for {
                          tunnel: w510 -> [w535] mode=indexing
                          tunnel: [w532] -> w503 mode=indexing
                          tunnel: [w531] -> w502 mode=indexing
                          n187 = Equal?(x=w535, y=timestamp(0 s since 1904-01-01)) -> (x = y?=w533:bool)
                          n188 = case shown="False" w533 {
                            tunnel: w535 -> [w541 _]
                            tunnel: [w537 "NaN"] -> w532
                            tunnel: [w536 "NaN"] -> w531
                            frame False {
                              n189 = property on="Graph Start Time" class="LVObjRef (strict)"() -> ("Value"=w546:refnum<vi>)  [unwired: 2 in, 2 out]
                              n190 = property class="AbsTime (strict)"(reference=w546) -> ("Value"=w544:timestamp)  [unwired: 1 in, 2 out]
                              n191 = To Double Precision Float(number=w541) -> (double precision float=w545:dbl)
                              n192 = To Double Precision Float(number=w544) -> (double precision float=w543:dbl)
                              n193 = Subtract(x=w545, y=w543) -> (x-y=w540:dbl)
                              n194 = Format Into String(format string="%<%H:%M:%S%3u %m/%d/%Y>T", w541) -> (resulting string=w537:string)  [unwired: 2 in, 1 out]
                              n195 = Number To Fractional String(number=w540, width (-)=i16 9, precision (6)=i16 3) -> (F-format string=w536:string)  [unwired: 1 in]
                            }
                            frame True {
                            }
                          }
                        }
                        n196 = Quotient & Remainder(x=w456, y=1) -> (x-y*floor(x/y)=w453:i32, floor(x/y)=w454:i32)
                        n197 = property on="QCM Graph" class="LVObjRef (strict)"() -> ("Value"=w520:refnum<vi>)  [unwired: 2 in, 2 out]
                        n198 = Equal To 0?(x=w453) -> (x = 0?=w452:bool)
                        n199 = And "Measure Rs?"(x=w452, y=TRUE) -> (x .and. y?=w450:bool)
                        n200 = property class="XYGraph (strict)"(reference=w520) -> ("Value"=w519:cluster{dbl[], dbl[]}[])  [unwired: 1 in, 2 out]
                        n201 = case shown="True" w450 {
                          tunnel: w454 -> [_ w525]
                          tunnel: [_ w522] -> w458
                          tunnel: [_ w521] -> w457
                          frame False {
                          }
                          frame True {
                            # "Keithley/ device control string"
                            # "Rows per cycle reads"
                            # "Current (A) used in vdP"
                            # "GPC value"
                            n202 = call "Resistivity_engine.vi"("I (A)"=0.001, "M"=1, "GPC (A/cycle)"=1.0, "N (cycle)"=w525, "Keithley 4200 VISA"=refnum<visa-resource-name> "TCPIP0::192.168.0.4::1225::SOCKET") -> ("error out"=w526:errorcluster, "rho (uOhm*cm)"=w523:dbl, "Rs (Ohm/sq)"=w524:dbl)  [unwired: 2 in, 2 out]
                            n203 = call <vilib>:"Clear Errors.vi"("error in (no error)"=w526) -> ()  [unwired: 5 in, 2 out]
                            n204 = Number To Exponential String(number=w523) -> (E-format string=w521:string)  [unwired: 3 in]
                            n205 = Number To Exponential String(number=w524) -> (E-format string=w522:string)  [unwired: 3 in]
                          }
                        }
                        n206 = Index Array(array=w519, index=0) -> (element=w517:cluster{dbl[], dbl[]})
                        n207 = Unbundle(w517) -> (w515:dbl[])  [unwired: 1 out]
                        n208 = Array Size(array=w515) -> (size(s)=w516:i32)
                        n209 = property on="Process Settings" class="LVObjRef (strict)"() -> ("Value"=w482:refnum<vi>)  [unwired: 2 in, 2 out]
                        n210 = Subtract(x=w516, y=10) -> (x-y=w513:i32)
                        n211 = property class="Clust (strict)"(reference=w482) -> ("Controls[]"=w481:refnum<vi>[])  [unwired: 1 in, 2 out]
                        n212 = Array Subset(array=w515, index=w513) -> (w512:dbl[])  [unwired: 1 in]
                        n213 = property on="InitialMass-i" class="DigNum (strict)"() -> ("Value"=w501:dbl)  [unwired: 2 in, 2 out]
                        n214 = call-poly <vilib>:"Mean.vi"("X"=w512) -> ("mean"=w500:dbl)  [unwired: 1 out]
                        "FinalMass-i" <- w500
                        n215 = Index Array(array=w481, index=0) -> (element=w479:refnum<vi>)
                        n216 = Subtract(x=w500, y=w501) -> (x-y=w499:dbl)
                        "DeltaM-i" <- w499
                        n217 = To More Specific Class(target class=w478, reference=w479) -> (specific class reference=w477:refnum<vi>)  [unwired: 1 in, 1 out]
                        n218 = property class="Ring"(reference=w477) -> ("Strings []"=w475:string[])  [unwired: 1 in, 2 out]
                        n219 = Build Array(w501, w500, w499) -> (w496:dbl[])
                        n220 = Number To Fractional String(number=w496, width (-)=i16 5, precision (6)=i16 0) -> (F-format string=w492:string[])  [unwired: 1 in]
                        n221 = property on="ProcessType-i" class="DigNum (strict)"() -> ("Value"=w473:i32)  [unwired: 2 in, 2 out]
                        n222 = property on="Precursor-i" class="DigNum (strict)"() -> ("Value"=w488:i32)  [unwired: 2 in, 2 out]
                        n223 = Build Array (concatenate)("0: Purge", w475) -> (w474:string[])
                        n224 = property on="Precursor-i name" class="Str"() -> ("Value"=w483:string)  [unwired: 2 in, 2 out]
                        n225 = Index Array(array=w503, index #1=0 ("index"), index #2=1 ("index"), index #3=2 ("index")) -> (element #1=w471:string, element #2=w469:string, element #3=w467:string)
                        n226 = Index Array(array=w502, index #1=0 ("index"), index #2=1 ("index"), index #3=2 ("index")) -> (element #1=w470:string, element #2=w468:string, element #3=w466:string)
                        n227 = Index Array(array=w492, index #1=0 ("index"), index #2=1 ("index"), index #3=2 ("index")) -> (element #1=w465:string, element #2=w464:string, element #3=w463:string)
                        n228 = Index Array(array=w474, index=w473) -> (element=w472:string)
                        n229 = Format Into String(w511) -> (resulting string=w485:string)  [unwired: 3 in, 1 out]
                        n230 = Number To Fractional String(number=w488, width (-)=i16 1, precision (6)=i16 0) -> (F-format string=w484:string)  [unwired: 1 in]
                        n231 = Build Array(w485, w484, w483, w472, w471, w470, w469, w468, w467, w466, w465, w464, w463, w458, w457) -> (w462:string[])
                        n232 = property on="Dose File Refnum" class="Ref (strict)"() -> (error out=w489:errorcluster, "Value"=w491:refnum<file>)  [unwired: 2 in, 1 out]
                        n233 = Array To Spreadsheet String(delimiter (Tab)="\t", array=w462, 3:"%s" ("format string")) -> (spreadsheet string=w459:string)
                        n234 = Write to Text File(file (use dialog)=w491, text=w459) -> (refnum out=w490:refnum<file>)  [unwired: 2 in, 2 out]
                        n235 = property on="Dose File Refnum" class="Ref (strict)"(error in=w489, "Value"=w490) -> ()  [unwired: 1 in, 2 out]
                      }
                      frame True {
                        # "If FileRefnum is not a refnum (i.e. Data Logging is off) do nothing"
                      }
                    }
                  }
                }
                n236 = Less Or Equal?(x=w287, y=4) -> (x <= y?=w293:bool)
                n237 = case shown="False" w293 {
                  tunnel: [w549 0 ("Column")] -> w294
                  tunnel: w287 -> [w551 _]
                  frame False {
                    n238 = Subtract(x=w551, y=4) -> (x-y=w549:i32)
                  }
                  frame True {
                  }
                }
                n239 = property on="Execution Table" class="LVObjRef (strict)"() -> ("Value"=w285:refnum<vi>)  [unwired: 2 in, 2 out]
                n240 = Bundle(w287, "Column"=-2) -> (w288:cluster{i32, "Column":i32})  [unwired: 1 in]
                n241 = Bundle("Column"=w294, "Column"=0) -> (w290:cluster{"Column":i32, "Column":i32})  [unwired: 1 in]
                n242 = property on="Property Node" class="Tbl (strict)"(reference=w285, "Active Cell"=w288, "Index Values"=w290, "Cell BG Color"=u32 6618880) -> ()  [unwired: 1 in, 2 out]
              }
              frame True {
                # "If the CheckAbortProcess subVI returns a true value, do nothing. \n(Note: CheckAbortProcess subVI returns a boolean true value that will stop loop execution and abort the process.)"
              }
            }
            n243 = Compound Arithmetic op=OR(w267, w266, w268) -> (w265:bool)
            "Total Steps" <- w232
          }
        }
      }
    }
    frame #2 {
      # "End ALD process, clean up."
      n244 = flat-sequence {
        tunnel: [w556] -> w555
        tunnel: w555 -> [w616]
        tunnel: [w614] -> w554
        tunnel: w554 -> [w633]
        frame #0 {
          n245 = property on="Dose File Refnum" class="Ref (strict)"() -> ("Value"=w559:refnum<file>)  [unwired: 2 in, 2 out]
          n246 = Equal?(x=w559, y=refnum<k0> refnum) -> (x = y?=w558:bool)
          n247 = case shown="False" w558 {
            tunnel: w559 -> [w595 _]
            tunnel: [w589 ""] -> w557
            frame False {
              # "If FileRefnum is a valid refnum (i.e. Data Logging is turned on), close the data file and alert user that data was successfully saved."
              n248 = Close File(refnum=w595) -> (path=w592:path, error out=w594:errorcluster)  [unwired: 1 in]
              n249 = Strip Path(path=w592) -> (stripped path=w591:path)  [unwired: 1 out]
              n250 = property on="Dose File Refnum" class="Ref (strict)"(error in=w594, "Value"=refnum<k0> refnum) -> ()  [unwired: 1 in, 2 out]
              n251 = Path To String(path=w591) -> (string=w588:string)
              n252 = Concatenate Strings(" Data and graphs saved to ", "\t", w588) -> (w589:string)
            }
            frame True {
              # "If FileRefnum is not a refnum (i.e. Data Logging is off) do nothing"
            }
          }
          n253 = property on="output cluster 4" class="Clust (strict)"() -> ("Value"=w568:T2)  [unwired: 2 in, 2 out]
          n254 = Unbundle By Name(w568) -> ("Execution Table"=w579:refnum<vi>, "Program Control"=w582:refnum<vi>, "Run ALD process"=w566:refnum<vi>, "ALD Process Running?"=w585:refnum<vi>)
          n255 = property on="output cluster" class="Clust (strict)"() -> ("Value"=w567:T3)  [unwired: 2 in, 2 out]
          n256 = Unbundle By Name(w567) -> ("Data Logging"=w571:refnum<vi>, "MFC Control"=w570:refnum<vi>, "QCM Control"=w569:refnum<vi>, "Process and Logging \nStatus Indicators"=w584:refnum<vi>)
          n257 = Unbundle By Name(w568) -> ("Module 7 \nValve Control"=w576:refnum<vi>, "Module 8 \nValve Control"=w575:refnum<vi>, "Process Settings"=w574:refnum<vi>, "Precursors"=w573:refnum<vi>, "CLEAR GRAPHS"=w572:refnum<vi>)
          n258 = Build Array(w576, w575, w574, w573, w572, w571, w570, w569) -> (w577:refnum<vi>[])
          n259 = property on="Property Node" class="Tbl (strict)"(reference=w579, "Active Cell"=T8 {"Row"=-2, "Column"=-2} ("Active Cell:Active Cell"), "Cell BG Color"=u32 16448250) -> (error out=w565:errorcluster)  [unwired: 1 in, 1 out]
          n260 = property on="Property Node" class="TabCtl (strict)"(reference=w582, "Value"=enum32{"Initialization", "ALD Recipe"}."ALD Recipe") -> (error out=w564:errorcluster)  [unwired: 1 in, 1 out]
          n261 = property on="Property Node" class="Bool (strict)"(reference=w566) -> (reference out=w586:refnum<vi>, error out=w563:errorcluster, "Value"=w562:bool)  [unwired: 1 in]
          n262 = call "SubVI_DisableControls_V16.vi"("appended array"=w577, "Disabled?"=FALSE) -> ("error out"=w561:errorcluster)  [unwired: 9 in]
          n263 = case shown="True" w562 {
            tunnel: w584 -> [w597 w613]
            tunnel: w586 -> [_ w612]
            tunnel: w585 -> [_ w611]
            tunnel: w565 -> [_ _]
            tunnel: w564 -> [_ _]
            tunnel: w563 -> [_ _]
            tunnel: w561 -> [_ _]
            tunnel: w557 -> [_ w610]
            tunnel: [w597 w602] -> w556
            frame False {
            }
            frame True {
              # "These clean-up tasks are only required if the process reached completion without being aborted (Run ALD Process is still true). If the process was aborted by the user or by the Pressure/Temp/MFC flow going out of range, the CheckAbortProcess subVI takes care of the below tasks."
              n264 = property on="Property Node" class="Bool (strict)"(reference=w612, "Value"=FALSE ("Run ALD process")) -> ()  [unwired: 1 in, 2 out]
              n265 = property class="Bool (strict)"(reference=w611, "Value"=FALSE) -> ()  [unwired: 1 in, 2 out]
              n266 = Concatenate Strings("ALD Process Complete." ("message"), w610) -> (w601:string)
              n267 = Get Date/Time In Seconds() -> (seconds since 1Jan1904=w600:timestamp)
              n268 = Format Into String(format string="%<%H:%M:%S%3u %m/%d/%Y>T", w600) -> (resulting string=w598:string)  [unwired: 2 in, 1 out]
              n269 = property class="Clust (strict)"(reference=w613) -> (reference out=w606:refnum<vi>, "Value"=w607:T13)  [unwired: 1 in, 1 out]
              n270 = Bundle By Name(cluster=w607, "Process End Time:"=w598, "Logging Data to:"=path "", "ALD Process Status:"=w601) -> (w608:T13)
              n271 = property class="Clust (strict)"(reference=w606, "Value"=w608) -> (reference out=w602:refnum<vi>)  [unwired: 1 in, 1 out]
            }
          }
        }
        frame #1 {
          n272 = property on="Summary File Refnum" class="Ref (strict)"() -> ("Value"=w617:refnum<file>)  [unwired: 2 in, 2 out]
          n273 = property class="Clust (strict)"(reference=w616) -> ("Value"=w615:T13)  [unwired: 1 in, 2 out]
          n274 = Equal?(x=w617, y=refnum<k0> refnum) -> (x = y?=w619:bool)
          n275 = case shown="False" w619 {
            tunnel: w617 -> [w630 _]
            tunnel: w615 -> [w620 _]
            frame False {
              w625 = "\r\n"
              w626 = "\t"
              # "If FileRefnum is a valid refnum (i.e. Data Logging is turned on), close the complete and close the summary file."
              n276 = Unbundle By Name(w620) -> ("Process End Time:"=w623:string, "Steps Completed:"=w622:string, "ALD Process Status:"=w621:string)
              n277 = Concatenate Strings("Process End Timestamp:" ("string"), w626, w623, w625, "Steps Completed:" ("string"), w626, w622, w625, w621, w625) -> (w624:string)
              n278 = Write to Text File(file (use dialog)=w630, text=w624) -> (refnum out=w629:refnum<file>)  [unwired: 2 in, 2 out]
              n279 = Close File(refnum=w629) -> (error out=w632:errorcluster)  [unwired: 1 in, 1 out]
              n280 = property on="Summary File Refnum" class="Ref (strict)"(error in=w632, "Value"=refnum<k0> refnum) -> ()  [unwired: 1 in, 2 out]
            }
            frame True {
              # "If FileRefnum is not a refnum (i.e. Data Logging is off) do nothing"
            }
          }
          n281 = Unbundle By Name(w615) -> ("ALD Process Status:"=w614:string)
        }
        frame #2 {
          n282 = One Button Dialog(message=w633) -> ()  [unwired: 1 in, 1 out]
        }
      }
    }
  }
  "error out" <- w1
